vi "Close.vi"(10 "VI":refnum<vi>) -> ()   [LabVIEW 2025, in "_Shared.lvlib" / "Panel.lvlib"]
uses:
  Panel.lvlib
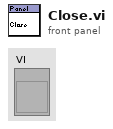
[diagram p1: front panel]
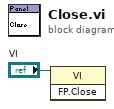
[diagram p0: block diagram]
diagram:
  n1 = invoke class="VI" method="FP.Close"(reference="VI") -> ()  [unwired: 2 in, 3 out]
